vi "Get Interpreter Info from Cluster.vi"(8 "error in":errorcluster, 11 "Host Initialization--cluster":T1) -> (0 "error out":errorcluster, 3 "IP:Port:Master/Slave":string)   [LabVIEW 2021, in "Common RT.lvlib"]
uses:
  Modules/Host/Host Interpreter/Host Initialization--cluster.ctl
  Common RT.lvlib
  UDP Comms/UDP Comms.lvlib
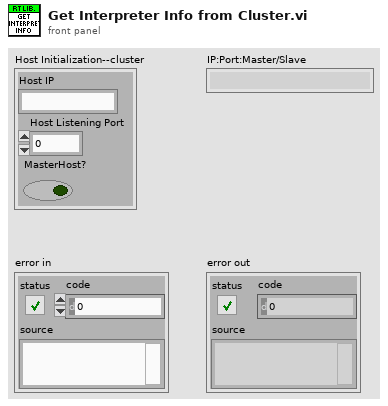
[diagram p1: front panel]
types:
  T1 = typedef "UDP Comms.lvlib/Host Initialization--cluster.ctl" = cluster{"Host IP":string, "Host Listening Port":u16, "MasterHost?":bool}
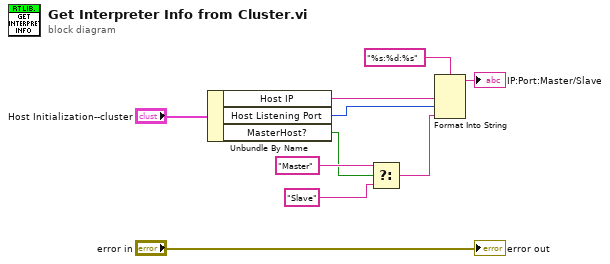
[diagram p0: block diagram]
diagram:
  n1 = Unbundle By Name("Host Initialization--cluster") -> ("Host IP"=w8:string, "Host Listening Port"=w7:u16, "MasterHost?"=w4:bool)
  n2 = Select(t="Master" ("format string"), s=w4, f="Slave" ("format string")) -> (s? t:f=w3:string)
  n3 = Format Into String(format string="%s:%d:%s", w8, w7, w3) -> (resulting string=→"IP:Port:Master/Slave":string)  [unwired: 2 in, 1 out]
  "error out" <- "error in"
